vi "Inject Fan Controller.vi"(7 "Fan Controller Ref":refnum<data-value>, 8 "error in (no error)":errorcluster, 11 "Stop Air Dry in":refnum<class "Stop Air Dry.lvclass">) -> (0 "error out":errorcluster, 3 "Stop Air Dry out":refnum<class "Stop Air Dry.lvclass">)   [LabVIEW 2019, in "Stop Air Dry.lvclass"]
uses:
  <vilib>/gpm_packages/@cs/Car-wash/Source/Process Steps/Stop Air Dry/Stop Air Dry.lvclass
  <vilib>/gpm_packages/@cs/Car-wash/Source/iFan Controller/iFan Controller.lvclass
  <vilib>/gpm_packages/@cs/Car-wash/Source/Process Steps/Stop Air Dry/Stop Air Dry.lvclass/Stop Air Dry.ctl
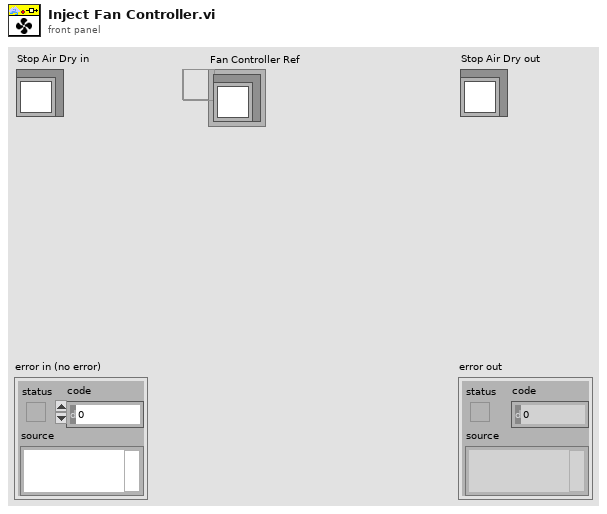
[diagram p1: front panel]
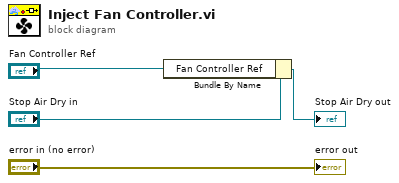
[diagram p0: block diagram]
diagram:
  n1 = Bundle By Name(cluster="Stop Air Dry in", "Fan Controller Ref"="Fan Controller Ref") -> (→"Stop Air Dry out":refnum<class "Stop Air Dry.lvclass">)
  "error out" <- "error in (no error)"
